vi "Populate Front Panel SLM.vi"(11 "This VI":refnum<vi>) -> ()   [LabVIEW 2014]
uses:
  TypeDefs/SLM Parameters.ctl
  <vilib>/vision/Image Controls.llb/IMAQ Image.ctl
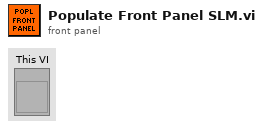
[diagram p1: front panel]
types:
  T1 = typedef "SLM Parameters.ctl" = cluster{"Error":errorcluster, "References":cluster{"Main VI":refnum<vi>, "SLM VI":refnum<vi>}, "Directories":cluster{"Root Directory":path, "Output Directory":path}, "Holo size":u16, "X pos":i16, "Y pos":i16, "Mode Coeffs":dbl[][], "Wrap Value":i32, "Lambda (nm)":dbl, "NA":dbl, "Base Name":string, "Win Num":i32, "SLM SN":string, "Holo Image Name":string, "Matrix Name":string, "Mode Matrix":dbl[][], "Flatness":u8[][], "STED Phase":dbl[][], "Ab Corr":dbl[][], "Holo Image":T2, "Holo Position":cluster{dbl, dbl, dbl, dbl}, "Apply Flatness\ncorr.?":bool, "Max Wavelength (nm)":dbl, "Min Wavelength (nm)":dbl, "Vortex Rotation":i16, "Top Hat Radius":dbl, "SLM ID Num":string, "Max Zernike Modes":i16, "Screen Width":i32, "Ab Corr VI":cluster{"AC VI Ref":refnum<vi>, "# Modes":i32, "Mode Array":dbl[][], "Apply Corr?":bool, "Step Size":dbl, "# Steps  ":u16, "Resolution":dbl, "FOV (um)":dbl, "Metric Images":dbl[][][][], "Metric Values":dbl[][], "S":dbl[], "I":dbl[], "M":dbl[], "Coeff Steps":dbl[], "Mode Loop":cluster{"Mode":i8, "Metric":i8, "Loop Index":i8}}}
  T2 = typedef "IMAQ Image.ctl" = refnum<image>
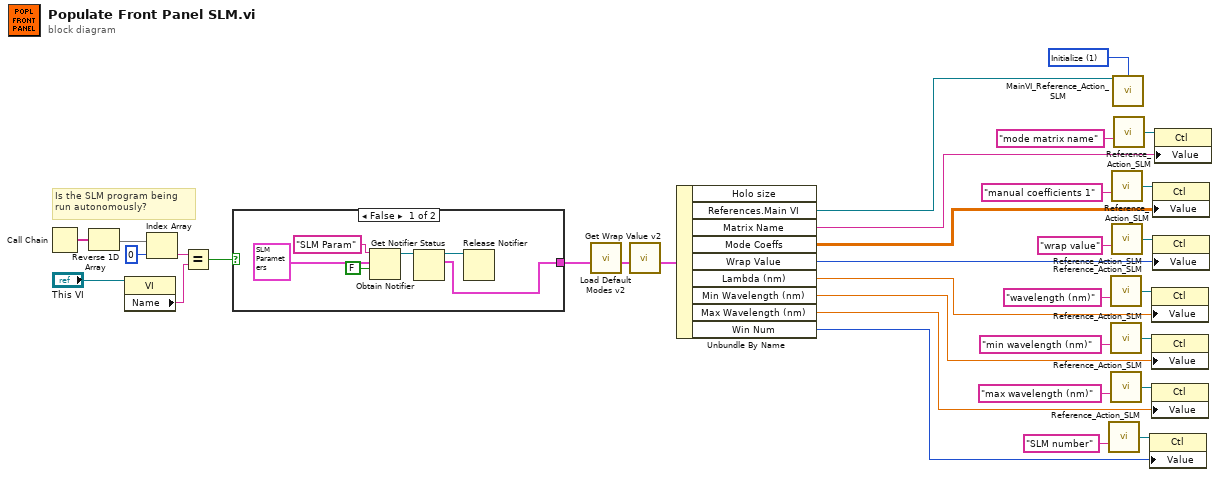
[diagram p0: block diagram]
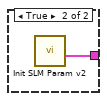
[diagram p2: hidden frame]
diagram:
  w1 = u16 1 items=["Read", "Initialize"] ("Action")
  # "Is the SLM program being \nrun autonomously?"
  n1 = Call Chain() -> (call chain=w13:string[])
  n2 = Reverse 1D Array(array=w13) -> (reversed array=w11:string[])
  n3 = property class="VI"(reference="This VI") -> ("Name"=w8:string)  [unwired: 1 in, 2 out]
  n4 = Index Array(array=w11, index=0) -> (element=w9:string)
  n5 = Equal?(x=w9, y=w8) -> (x = y?=w10:bool)
  n6 = case shown="False" w10 {
    tunnel: [w34 w40] -> w7
    frame False {
      n7 = Obtain Notifier(name (unnamed)="SLM Param", notification data type=T1 {"Error"={"status"=FALSE, "code"=0, "source"=""}, "References"={"Main VI"=refnum, "SLM VI"=refnum}, "Directories"={"Root Directory"=path "C:/Documents and Settings/tg273/My Documents/LabView VIs/Yale SLM/Yale v2/Mode Matrices", "Output Directory"=path "C:/Documents and Settings/tg273/My Documents/LabView VIs/Yale SLM/Yale v2/Mode Matrices"}, "Holo size"=504, "X pos"=-3, "Y pos"=-40, "Mode Coeffs"=[[2.0, 0.0], [3.0, 18.0], [4.0, 0.0], [11.0, 0.0], [22.0, 0.0], [37.0, 0.0], [5.0, 0.0], [6.0, 0.0], [7.0, 0.0], [8.0, 0.0], [9.0, 0.0], [10.0, 0.0]], "Wrap Value"=197, "Lambda (nm)"=750.0, "NA"=1.4, "Base Name"="", "Win Num"=2, "SLM SN"="0600535", "Holo Image Name"="0600535", "Matrix Name"="Unit Matrix.csv", "Mode Matrix"=array36x36[1296 elements], "Flatness"=array600x792[475200 elements], "STED Phase"=array504x504[254016 elements], "Ab Corr"=array504x504[254016 elements], "Holo Image"="remote image 000000000731AF64", "Holo Position"={-3.0, -40.0, 3840.0, 504.0}, "Apply Flatness\ncorr.?"=TRUE, "Max Wavelength (nm)"=750.0, "Min Wavelength (nm)"=750.0, "Vortex Rotation"=-3, "Top Hat Radius"=1.4, "SLM ID Num"="0600535", "Max Zernike Modes"=-3, "Screen Width"=2, "Ab Corr VI"={"AC VI Ref"=refnum, "# Modes"=0, "Mode Array"=[], "Apply Corr?"=FALSE, "Step Size"=0.0, "# Steps  "=0, "Resolution"=0.0, "FOV (um)"=0.0, "Metric Images"=[], "Metric Values"=[], "S"=[], "I"=[], "M"=[], "Coeff Steps"=[], "Mode Loop"={"Mode"=0, "Metric"=0, "Loop Index"=0}}} ("SLM Parameters"), create if not found? (T)=FALSE) -> (notifier out=w37:refnum<notifier>)  [unwired: 1 in, 2 out]
      n8 = Get Notifier Status(notifier=w37) -> (notifier out=w39:refnum<notifier>, current notification=w34:T1)  [unwired: 1 in, 3 out]
      n9 = Release Notifier(notifier=w39) -> ()  [unwired: 2 in, 3 out]
    }
    frame True {
      n10 = call "Init SLM Param v2.vi"() -> ("SLM Param Out"=w40:T1)  [unwired: 11 in]
    }
  }
  n11 = call "Load Default Modes v2.vi"("SLM Param In"=w7) -> ("SLM Param Out"=w33:T1)  [unwired: 10 in]
  n12 = call "Get Wrap Value v2.vi"("SLM Param In"=w33) -> ("SLM Param Out"=w32:T1)  [unwired: 10 in]
  n13 = Unbundle By Name(w32) -> ("References.Main VI"=w2:refnum<vi>, "Matrix Name"=w4:string, "Mode Coeffs"=w26:dbl[][], "Wrap Value"=w29:i32, "Lambda (nm)"=w23:dbl, "Min Wavelength (nm)"=w18:dbl, "Max Wavelength (nm)"=w17:dbl, "Win Num"=w14:i32)  [unwired: 1 out]
  n14 = call "Reference_Action_SLM.vi"("Control Name"="SLM number") -> ("Ref OUT"=w15:refnum<vi>)  [unwired: 12 in, 2 out]
  n15 = call "Reference_Action_SLM.vi"("Control Name"="wavelength (nm)") -> ("Ref OUT"=w25:refnum<vi>)  [unwired: 12 in, 2 out]
  n16 = call "Reference_Action_SLM.vi"("Control Name"="min wavelength (nm)") -> ("Ref OUT"=w20:refnum<vi>)  [unwired: 12 in, 2 out]
  n17 = call "Reference_Action_SLM.vi"("Control Name"="max wavelength (nm)") -> ("Ref OUT"=w19:refnum<vi>)  [unwired: 12 in, 2 out]
  n18 = call "Reference_Action_SLM.vi"("Control Name"="manual coefficients 1") -> ("Ref OUT"=w28:refnum<vi>)  [unwired: 12 in, 2 out]
  n19 = call "Reference_Action_SLM.vi"("Control Name"="wrap value") -> ("Ref OUT"=w31:refnum<vi>)  [unwired: 12 in, 2 out]
  n20 = call "MainVI_Reference_Action_SLM.vi"("VI Ref IN"=w2, "Action"=w1) -> ()  [unwired: 13 in, 1 out]
  n21 = call "Reference_Action_SLM.vi"("Control Name"="mode matrix name") -> ("Ref OUT"=w6:refnum<vi>)  [unwired: 12 in, 2 out]
  n22 = property class="Ctl"(reference=w15, "Value"=w14) -> ()  [unwired: 1 in, 2 out]
  n23 = property class="Ctl"(reference=w25, "Value"=w23) -> ()  [unwired: 1 in, 2 out]
  n24 = property class="Ctl"(reference=w20, "Value"=w18) -> ()  [unwired: 1 in, 2 out]
  n25 = property class="Ctl"(reference=w19, "Value"=w17) -> ()  [unwired: 1 in, 2 out]
  n26 = property class="Ctl"(reference=w28, "Value"=w26) -> ()  [unwired: 1 in, 2 out]
  n27 = property class="Ctl"(reference=w31, "Value"=w29) -> ()  [unwired: 1 in, 2 out]
  n28 = property class="Ctl"(reference=w6, "Value"=w4) -> ()  [unwired: 1 in, 2 out]
